vi "Test IV and Ic distribution V3.vi"() -> ()   [LabVIEW 2024]
uses:
  RT fast data.ctl
  <vilib>/LabVIEW Targets/FPGA/cRIO/shared/nicrio_ModuleControls/nicrio_cRIO-9775_RecordDataRates4ChansRing.ctl
  <vilib>/LabVIEW Targets/FPGA/cRIO/shared/nicrio_ModuleControls/nicrio_BasicConversionTime.ctl
  Ramps.ctl
  <resource>/objmgr/ni.dex.rc
  <vilib>/Analysis/NI_AALBase.lvlib
panel:
  in  "Tab Control 2":T1(tab)=enum."Ic distribution"
  out "IV":cluster{"Y":dbl[], "Y":dbl[]}[](graph)
  out "Waveform Graph":dbl[][](graph)
  out "Histogram Graph":T2(graph)={"X Values"=[4.536339111328125, 4.540169677734375, 4.544000244140625, 4.547830810546874, 4.551661376953124, 4.555491943359374, 4.559322509765623, 4.563153076171873, 4.566983642578123, 4.570814208984372, 4.574644775390622, 4.578475341796872, 4.5823059082031214, 4.586136474609371, 4.589967041015621, 4.5937976074218705, 4.59762817382812, 4.60145874023437, 4.6052893066406195, 4.609119873046869, 4.612950439453119, 4.616781005859369, 4.620611572265618, 4.624442138671868, 4.628272705078118, 4.632103271484367, 4.635933837890617, 4.639764404296867, 4.643594970703116, 4.647425537109366, 4.651256103515616, 4.655086669921865, 4.658917236328115, 4.662747802734365, 4.666578369140614, 4.670408935546864, 4.674239501953114, 4.6780700683593635, 4.681900634765613, 4.685731201171863, 4.6895617675781125, 4.693392333984362, 4.697222900390612, 4.7010534667968615, 4.704884033203111, 4.708714599609361, 4.712545166015611, 4.71637573242186, 4.72020629882811, 4.72403686523436, 4.727867431640609, 4.731697998046859, 4.735528564453109, 4.739359130859358, 4.743189697265608, 4.747020263671858, 4.750850830078107, 4.754681396484357, 4.758511962890607, 4.762342529296856, 4.766173095703106, 4.770003662109356, 4.7738342285156055, 4.777664794921855, 4.781495361328105, 4.7853259277343545, 4.789156494140604, 4.792987060546854, 4.7968176269531035, 4.800648193359353, 4.804478759765603, 4.808309326171853, 4.812139892578102, 4.815970458984352, 4.819801025390602, 4.823631591796851, 4.827462158203101, 4.831292724609351, 4.8351232910156, 4.83895385742185, 4.8427844238281, 4.846614990234349, 4.850445556640599, 4.854276123046849, 4.858106689453098, 4.861937255859348, 4.865767822265598, 4.8695983886718475, 4.873428955078097, 4.877259521484347, 4.8810900878905965, 4.884920654296846, 4.888751220703096, 4.8925817871093455, 4.896412353515595, 4.900242919921845, 4.904073486328095, 4.907904052734344, 4.911734619140594, 4.915565185546844], "Histogram: h(x)"=[1, 2, 2, 2, 0, 2, 1, 2, 0, 2, 2, 1, 2, 4, 4, 2, 1, 3, 3, 4, 7, 5, 12, 12, 10, 8, 15, 8, 14, 9, 6, 10, 12, 16, 9, 11, 30, 17, 15, 28, 22, 14, 24, 13, 25, 23, 23, 19, 28, 18, 21, 14, 32, 36, 18, 28, 8, 18, 22, 21, 21, 8, 22, 19, 8, 8, 16, 12, 12, 5, 18, 15, 6, 17, 5, 9, 4, 7, 5, 4, 7, 6, 3, 10, 5, 4, 7, 0, 0, 2, 1, 4, 3, 2, 1, 0, 0, 0, 2, 1]}
  in  "intervals":i32=100
  in  "Tab Control":T3(tab)=enum."Ic"
  in  "cRIO IP":string="//172.22.11.2"
  in  "Data buffer size":i32=1000
  in  "IV parameters":T4={"Records Num"=1, "AI Trigger Configuration"={"Trigger Slope"=enum."Positive", "Trigger Level"=0.89990234375, "Hystesis Value"=0.0, "AI Channel"=0}, "Record PreTrigger Samples"=1, "Record Samples"=2300, "Ic Cut off or curve"=FALSE, "Record Data Rate"=200, "Wait before trigger us"=0, "Cutoff delay usec"=0, "Timing Mode"=enum."High Resolution", "Trigger length ticks"=1, "Timeout"=-1, "Ramps"={"Amp"=8.0, "Delay time 10us"=1000, "Ramp1 time 10us"=1000, "Ramp2 time 10us"=200, "Ramp3 time 10us"=100, "End time 10us"=0}} {"Record Data Rate" items=["20.000 MS/s (NI 9775)"=1, "10.00 MS/s (NI 9775)"=2, "6.667 MS/s (NI 9775)"=3, "5.000 MS/s (NI 9775)"=4, "2.500 MS/s (NI 9775)"=8, "1.667 MS/s (NI 9775)"=12, "1.250 MS/s (NI 9775)"=16, "1.000 MS/s (NI 9775)"=20, "833.333 KS/s (NI 9775)"=24, "714.286 KS/s (NI 9775)"=28, "625.000 KS/s (NI 9775)"=32, "555.556 KS/s (NI 9775)"=36, "500.000 KS/s (NI 9775)"=40, "454.545 KS/s (NI 9775)"=44, "416.667 KS/s (NI 9775)"=48, "384.615 KS/s (NI 9775)"=52, "357.143 KS/s (NI 9775)"=56, "333.333 KS/s (NI 9775)"=60, "312.500 KS/s (NI 9775)"=64, "294.118 KS/s (NI 9775)"=68, "277.778 KS/s (NI 9775)"=72, "263.158 KS/s (NI 9775)"=76, "250.000 KS/s (NI 9775)"=80, "238.095 KS/s (NI 9775)"=84, "227.273 KS/s (NI 9775)"=88, "217.391 KS/s (NI 9775)"=92, "208.333 KS/s (NI 9775)"=96, "200.000 KS/s (NI 9775)"=100, "192.308 KS/s (NI 9775)"=104, "185.185 KS/s (NI 9775)"=108, "178.571 KS/s (NI 9775)"=112, "172.414 KS/s (NI 9775)"=116, "166.667 KS/s (NI 9775)"=120, "161.290 KS/s (NI 9775)"=124, "156.250 KS/s (NI 9775)"=128, "151.515 KS/s (NI 9775)"=132, "147.059 KS/s (NI 9775)"=136, "142.857 KS/s (NI 9775)"=140, "138.889 KS/s (NI 9775)"=144, "135.135 KS/s (NI 9775)"=148, "131.579 KS/s (NI 9775)"=152, "128.205 KS/s (NI 9775)"=156, "125.000 KS/s (NI 9775)"=160, "121.951 KS/s (NI 9775)"=164, "119.048 KS/s (NI 9775)"=168, "116.279 KS/s (NI 9775)"=172, "113.636 KS/s (NI 9775)"=176, "111.111 KS/s (NI 9775)"=180, "108.696 KS/s (NI 9775)"=184, "106.383 KS/s (NI 9775)"=188, "104.167 KS/s (NI 9775)"=192, "102.041 KS/s (NI 9775)"=196, "100.000 KS/s (NI 9775)"=200, "50.000 KS/s (NI 9775)"=400, "33.333 KS/s (NI 9775)"=600, "25.000 KS/s (NI 9775)"=800, "20.000 KS/s (NI 9775)"=1000, "16.667 KS/s (NI 9775)"=1200, "14.286 KS/s (NI 9775)"=1400, "12.500 KS/s (NI 9775)"=1600, "11.111 KS/s (NI 9775)"=1800, "10.000 KS/s (NI 9775)"=2000, "9.091 KS/s (NI 9775)"=2200, "8.333 KS/s (NI 9775)"=2400, "7.692 KS/s (NI 9775)"=2600, "7.143 KS/s (NI 9775)"=2800, "6.667 KS/s (NI 9775)"=3000, "6.250 KS/s (NI 9775)"=3200, "5.882 KS/s (NI 9775)"=3400, "5.556 KS/s (NI 9775)"=3600, "5.000 KS/s (NI 9775)"=4000, "4.762 KS/s (NI 9775)"=4200, "4.545 KS/s (NI 9775)"=4400, "4.348 KS/s (NI 9775)"=4600, "4.167 KS/s (NI 9775)"=4800, "4.000 KS/s (NI 9775)"=5000, "3.846 KS/s (NI 9775)"=5200, "3.571 KS/s (NI 9775)"=5600, "3.333 KS/s (NI 9775)"=6000, "3.125 KS/s (NI 9775)"=6400, "2.941 KS/s (NI 9775)"=6800, "2.778 KS/s (NI 9775)"=7200, "2.632 KS/s (NI 9775)"=7600, "2.500 KS/s (NI 9775)"=8000, "2.381 KS/s (NI 9775)"=8400, "2.273 KS/s (NI 9775)"=8800, "2.174 KS/s (NI 9775)"=9200, "2.083 KS/s (NI 9775)"=9600, "2.000 KS/s (NI 9775)"=10000, "1.923 KS/s (NI 9775)"=10400, "1.852 KS/s (NI 9775)"=10800, "1.786 KS/s (NI 9775)"=11200, "1.724 KS/s (NI 9775)"=11600, "1.667 KS/s (NI 9775)"=12000, "1.613 KS/s (NI 9775)"=12400, "1.563 KS/s (NI 9775)"=12800, "1.515 KS/s (NI 9775)"=13200, "1.471 KS/s (NI 9775)"=13600, "1.429 KS/s (NI 9775)"=14000, "1.389 KS/s (NI 9775)"=14400, "1.351 KS/s (NI 9775)"=14800, "1.316 KS/s (NI 9775)"=15200, "1.282 KS/s (NI 9775)"=15600, "1.250 KS/s (NI 9775)"=16000, "1.220 KS/s (NI 9775)"=16400, "1.190 KS/s (NI 9775)"=16800, "1.163 KS/s (NI 9775)"=17200, "1.136 KS/s (NI 9775)"=17600, "1.111 KS/s (NI 9775)"=18000, "1.087 KS/s (NI 9775)"=18400, "1.064 KS/s (NI 9775)"=18800, "1.042 KS/s (NI 9775)"=19200, "1.020 KS/s (NI 9775)"=19600, "1.000 KS/s (NI 9775)"=20000, "0.980 KS/s (NI 9775)"=20400, "0.962 KS/s (NI 9775)"=20800, "0.943 KS/s (NI 9775)"=21200, "0.926 KS/s (NI 9775)"=21600, "0.909 KS/s (NI 9775)"=22000, "0.893 KS/s (NI 9775)"=22400, "0.877 KS/s (NI 9775)"=22800, "0.862 KS/s (NI 9775)"=23200, "0.847 KS/s (NI 9775)"=23600, "0.833 KS/s (NI 9775)"=24000, "0.820 KS/s (NI 9775)"=24400, "0.806 KS/s (NI 9775)"=24800, "0.794 KS/s (NI 9775)"=25200, "0.781 KS/s (NI 9775)"=25600, "0.694 KS/s (NI 9775)"=28800, "0.625 KS/s (NI 9775)"=32000, "0.568 KS/s (NI 9775)"=35200, "0.521 KS/s (NI 9775)"=38400, "0.446 KS/s (NI 9775)"=44800, "0.391 KS/s (NI 9775)"=51200, "0.347 KS/s (NI 9775)"=57600, "0.313 KS/s (NI 9775)"=64000]}
  in  "Ic parameters":T4={"Records Num"=1000, "AI Trigger Configuration"={"Trigger Slope"=enum."Positive", "Trigger Level"=0.199951171875, "Hystesis Value"=0.0, "AI Channel"=0}, "Record PreTrigger Samples"=1, "Record Samples"=16, "Ic Cut off or curve"=TRUE, "Record Data Rate"=1, "Wait before trigger us"=10000, "Cutoff delay usec"=0, "Timing Mode"=enum."High Resolution", "Trigger length ticks"=1, "Timeout"=-1, "Ramps"={"Amp"=8.0, "Delay time 10us"=1000, "Ramp1 time 10us"=1000, "Ramp2 time 10us"=200, "Ramp3 time 10us"=100, "End time 10us"=0}} {"Record Data Rate" items=["20.000 MS/s (NI 9775)"=1, "10.00 MS/s (NI 9775)"=2, "6.667 MS/s (NI 9775)"=3, "5.000 MS/s (NI 9775)"=4, "2.500 MS/s (NI 9775)"=8, "1.667 MS/s (NI 9775)"=12, "1.250 MS/s (NI 9775)"=16, "1.000 MS/s (NI 9775)"=20, "833.333 KS/s (NI 9775)"=24, "714.286 KS/s (NI 9775)"=28, "625.000 KS/s (NI 9775)"=32, "555.556 KS/s (NI 9775)"=36, "500.000 KS/s (NI 9775)"=40, "454.545 KS/s (NI 9775)"=44, "416.667 KS/s (NI 9775)"=48, "384.615 KS/s (NI 9775)"=52, "357.143 KS/s (NI 9775)"=56, "333.333 KS/s (NI 9775)"=60, "312.500 KS/s (NI 9775)"=64, "294.118 KS/s (NI 9775)"=68, "277.778 KS/s (NI 9775)"=72, "263.158 KS/s (NI 9775)"=76, "250.000 KS/s (NI 9775)"=80, "238.095 KS/s (NI 9775)"=84, "227.273 KS/s (NI 9775)"=88, "217.391 KS/s (NI 9775)"=92, "208.333 KS/s (NI 9775)"=96, "200.000 KS/s (NI 9775)"=100, "192.308 KS/s (NI 9775)"=104, "185.185 KS/s (NI 9775)"=108, "178.571 KS/s (NI 9775)"=112, "172.414 KS/s (NI 9775)"=116, "166.667 KS/s (NI 9775)"=120, "161.290 KS/s (NI 9775)"=124, "156.250 KS/s (NI 9775)"=128, "151.515 KS/s (NI 9775)"=132, "147.059 KS/s (NI 9775)"=136, "142.857 KS/s (NI 9775)"=140, "138.889 KS/s (NI 9775)"=144, "135.135 KS/s (NI 9775)"=148, "131.579 KS/s (NI 9775)"=152, "128.205 KS/s (NI 9775)"=156, "125.000 KS/s (NI 9775)"=160, "121.951 KS/s (NI 9775)"=164, "119.048 KS/s (NI 9775)"=168, "116.279 KS/s (NI 9775)"=172, "113.636 KS/s (NI 9775)"=176, "111.111 KS/s (NI 9775)"=180, "108.696 KS/s (NI 9775)"=184, "106.383 KS/s (NI 9775)"=188, "104.167 KS/s (NI 9775)"=192, "102.041 KS/s (NI 9775)"=196, "100.000 KS/s (NI 9775)"=200, "50.000 KS/s (NI 9775)"=400, "33.333 KS/s (NI 9775)"=600, "25.000 KS/s (NI 9775)"=800, "20.000 KS/s (NI 9775)"=1000, "16.667 KS/s (NI 9775)"=1200, "14.286 KS/s (NI 9775)"=1400, "12.500 KS/s (NI 9775)"=1600, "11.111 KS/s (NI 9775)"=1800, "10.000 KS/s (NI 9775)"=2000, "9.091 KS/s (NI 9775)"=2200, "8.333 KS/s (NI 9775)"=2400, "7.692 KS/s (NI 9775)"=2600, "7.143 KS/s (NI 9775)"=2800, "6.667 KS/s (NI 9775)"=3000, "6.250 KS/s (NI 9775)"=3200, "5.882 KS/s (NI 9775)"=3400, "5.556 KS/s (NI 9775)"=3600, "5.000 KS/s (NI 9775)"=4000, "4.762 KS/s (NI 9775)"=4200, "4.545 KS/s (NI 9775)"=4400, "4.348 KS/s (NI 9775)"=4600, "4.167 KS/s (NI 9775)"=4800, "4.000 KS/s (NI 9775)"=5000, "3.846 KS/s (NI 9775)"=5200, "3.571 KS/s (NI 9775)"=5600, "3.333 KS/s (NI 9775)"=6000, "3.125 KS/s (NI 9775)"=6400, "2.941 KS/s (NI 9775)"=6800, "2.778 KS/s (NI 9775)"=7200, "2.632 KS/s (NI 9775)"=7600, "2.500 KS/s (NI 9775)"=8000, "2.381 KS/s (NI 9775)"=8400, "2.273 KS/s (NI 9775)"=8800, "2.174 KS/s (NI 9775)"=9200, "2.083 KS/s (NI 9775)"=9600, "2.000 KS/s (NI 9775)"=10000, "1.923 KS/s (NI 9775)"=10400, "1.852 KS/s (NI 9775)"=10800, "1.786 KS/s (NI 9775)"=11200, "1.724 KS/s (NI 9775)"=11600, "1.667 KS/s (NI 9775)"=12000, "1.613 KS/s (NI 9775)"=12400, "1.563 KS/s (NI 9775)"=12800, "1.515 KS/s (NI 9775)"=13200, "1.471 KS/s (NI 9775)"=13600, "1.429 KS/s (NI 9775)"=14000, "1.389 KS/s (NI 9775)"=14400, "1.351 KS/s (NI 9775)"=14800, "1.316 KS/s (NI 9775)"=15200, "1.282 KS/s (NI 9775)"=15600, "1.250 KS/s (NI 9775)"=16000, "1.220 KS/s (NI 9775)"=16400, "1.190 KS/s (NI 9775)"=16800, "1.163 KS/s (NI 9775)"=17200, "1.136 KS/s (NI 9775)"=17600, "1.111 KS/s (NI 9775)"=18000, "1.087 KS/s (NI 9775)"=18400, "1.064 KS/s (NI 9775)"=18800, "1.042 KS/s (NI 9775)"=19200, "1.020 KS/s (NI 9775)"=19600, "1.000 KS/s (NI 9775)"=20000, "0.980 KS/s (NI 9775)"=20400, "0.962 KS/s (NI 9775)"=20800, "0.943 KS/s (NI 9775)"=21200, "0.926 KS/s (NI 9775)"=21600, "0.909 KS/s (NI 9775)"=22000, "0.893 KS/s (NI 9775)"=22400, "0.877 KS/s (NI 9775)"=22800, "0.862 KS/s (NI 9775)"=23200, "0.847 KS/s (NI 9775)"=23600, "0.833 KS/s (NI 9775)"=24000, "0.820 KS/s (NI 9775)"=24400, "0.806 KS/s (NI 9775)"=24800, "0.794 KS/s (NI 9775)"=25200, "0.781 KS/s (NI 9775)"=25600, "0.694 KS/s (NI 9775)"=28800, "0.625 KS/s (NI 9775)"=32000, "0.568 KS/s (NI 9775)"=35200, "0.521 KS/s (NI 9775)"=38400, "0.446 KS/s (NI 9775)"=44800, "0.391 KS/s (NI 9775)"=51200, "0.347 KS/s (NI 9775)"=57600, "0.313 KS/s (NI 9775)"=64000]}
  in  "Read point":i32=1
  out "DAQ_CMD_Writer endpoint":refnum<k21>="DAQ_CMD_Writer"
  out "PCreaderI":refnum<k21>="PCreaderI"
  out "PC para writer":refnum<k21>="PCwriter"
  out "DAQ_AI_Reader endpoint":refnum<k21>="DAQ_AI_Reader"
  out "PCreaderV":refnum<k21>="PCreaderV"
  out "error out":errorcluster
  in  "IV length":i32=7500
  in  "IV points start":i32
  out "Time to Init ms":u32=654
  out "Start time ms":u32=3519849804
  in  "Wire resistance":dbl
  out "Done":bool=TRUE
  out "Ic data":dbl[](array[numeric])=[4.69482421875, 4.79443359375, 4.6962890625, 4.82763671875, 4.8427734375, 4.723876953125, 4.7529296875, 4.690673828125, 4.736328125, 4.703125, 4.708740234375, 4.690673828125, 4.791748046875, 4.682373046875, 4.658935546875, 4.798583984375, 4.677001953125, 4.766845703125, 4.741943359375, 4.710205078125, 4.70458984375, 4.718505859375, 4.72802734375, 4.74462890625, 4.757080078125, 4.732177734375, 4.669921875, 4.77783203125, 4.791748046875, 4.740478515625, 4.712890625, 4.802734375, 4.6728515625, 4.710205078125, 4.6962890625, 4.748779296875, 4.7060546875, 4.747314453125, 4.77783203125, 4.6962890625, 4.7294921875, 4.698974609375, 4.7294921875, 4.562255859375, 4.68798828125, 4.610595703125, 4.717041015625, 4.689453125, 4.708740234375, 4.76806640625, 4.67822265625, 4.58154296875, 4.732177734375, 4.7060546875, 4.772216796875, 4.758544921875, 4.772216796875, 4.8525390625, 4.802734375, 4.733642578125, 4.83447265625, 4.8291015625, 4.805419921875, 4.6533203125, 4.69775390625, 4.7626953125, 4.67822265625, 4.72119140625, 4.73486328125, 4.71142578125, 4.75146484375, 4.823486328125, 4.766845703125, 4.755615234375, 4.718505859375, 4.805419921875, 4.773681640625, 4.8330078125, 4.80419921875, 4.72119140625, 4.815185546875, 4.802734375, 4.806884765625, 4.76806640625, 4.91064453125, 4.788818359375, 4.816650390625, 4.806884765625, 4.712890625, 4.758544921875, 4.718505859375, 4.826171875, 4.808349609375, 4.788818359375, 4.732177734375, 4.710205078125, 4.80419921875, 4.763916015625, 4.8095703125, 4.78466796875, 4.780517578125, 4.7294921875, 4.71435546875, 4.736328125, 4.747314453125, 4.779296875, 4.855224609375, 4.78466796875, 4.715576171875, 4.740478515625, 4.7431640625, 4.7763671875, 4.855224609375, 4.741943359375, 4.73486328125, 4.759765625, 4.763916015625, 4.759765625, 4.748779296875, 4.80126953125, 4.77099609375, 4.733642578125, 4.72119140625, 4.73486328125, 4.707275390625, 4.665771484375, 4.69482421875, 4.808349609375, 4.736328125, 4.72802734375, 4.7294921875, 4.765380859375, 4.779296875, 4.750244140625, 4.779296875, 4.65625, 4.668701171875, 4.772216796875, 4.747314453125, 4.723876953125, 4.8857421875, 4.682373046875, 4.71142578125, 4.781982421875, 4.70458984375, 4.77783203125, 4.8291015625, 4.81787109375, 4.7265625, 4.798583984375, 4.8125, 4.8330078125, 4.730712890625, 4.6865234375, 4.808349609375, 4.73779296875, 4.75439453125, 4.78466796875, 4.712890625, 4.790283203125, 4.7294921875, 4.715576171875, 4.736328125, 4.766845703125, 4.723876953125, 4.88427734375, 4.750244140625, 4.715576171875, 4.68115234375, 4.625732421875, 4.69775390625, 4.8193359375, 4.78759765625, 4.740478515625, 4.758544921875, 4.62841796875, 4.632568359375, 4.6796875, 4.7294921875, 4.755615234375, 4.74609375, 4.700439453125, 4.775146484375, 4.725341796875, 4.775146484375, 4.775146484375, 4.669921875, 4.685302734375, 4.70458984375, 4.88427734375, 4.765380859375, 4.717041015625, 4.701904296875, 4.73486328125, 4.75439453125, 4.6533203125, 4.63818359375, 4.6796875, 4.732177734375, 4.675537109375, 4.722412109375, 4.717041015625, 4.733642578125, 4.710205078125, 4.68115234375, 4.72119140625, 4.763916015625, 4.77783203125, 4.68798828125, 4.78466796875, 4.747314453125, 4.73779296875, 4.822021484375, 4.846923828125, 4.859375, 4.733642578125, 4.71435546875, 4.8095703125, 4.855224609375, 4.750244140625, 4.698974609375, 4.739013671875, 4.708740234375, 4.7529296875, 4.718505859375, 4.7431640625, 4.683837890625, 4.685302734375, 4.64501953125, 4.71142578125, 4.81787109375, 4.74609375, 4.730712890625, 4.81103515625, 4.748779296875, 4.682373046875, 4.73779296875, 4.755615234375, 4.66162109375, 4.682373046875, 4.690673828125, 4.77783203125, 4.759765625, 4.76806640625, 4.689453125, 4.8095703125, 4.715576171875, 4.710205078125, 4.6962890625, 4.61474609375, 4.75439453125, 4.617431640625, 4.625732421875, 4.73486328125, 4.62841796875, 4.635498046875, 4.75146484375, 4.74462890625, 4.700439453125, 4.763916015625, 4.66455078125, 4.82080078125, 4.6865234375, 4.765380859375, 4.7431640625, 4.757080078125, 4.7958984375, 4.765380859375, 4.758544921875, 4.690673828125, 4.68798828125, 4.685302734375, 4.74609375, 4.682373046875, 4.70458984375, 4.739013671875, 4.773681640625, 4.674072265625, 4.69482421875, 4.7265625, 4.6728515625, 4.69482421875, 4.76806640625, 4.72802734375, 4.824951171875, 4.7197265625, 4.66162109375, 4.765380859375, 4.71435546875, 4.76123046875, 4.6865234375, 4.750244140625, 4.73779296875, 4.74609375, 4.627197265625, 4.6865234375, 4.736328125, 4.73486328125, 4.723876953125, 4.74462890625, 4.76123046875, 4.587158203125, 4.7060546875, 4.693603515625, 4.73779296875, 4.69775390625, 4.70458984375, 4.72119140625, 4.70458984375, 4.733642578125, 4.6630859375, 4.717041015625, 4.7197265625, 4.864990234375, 4.84130859375, 4.708740234375, 4.701904296875, 4.748779296875, 4.740478515625, 4.775146484375, 4.710205078125, 4.775146484375, 4.750244140625, 4.675537109375, 4.7529296875, 4.74462890625, 4.741943359375, 4.718505859375, 4.6201171875, 4.7197265625, 4.76123046875, 4.755615234375, 4.788818359375, 4.7626953125, 4.816650390625, 4.715576171875, 4.76953125, 4.8525390625, 4.8427734375, 4.80419921875, 4.831787109375, 4.82080078125, 4.8359375, 4.802734375, 4.859375, 4.802734375, 4.773681640625, 4.815185546875, 4.758544921875, 4.89111328125, 4.856689453125, 4.781982421875, 4.848388671875, 4.848388671875, 4.86767578125, 4.91748046875, 4.808349609375, 4.757080078125, 4.798583984375, 4.755615234375, 4.889892578125, 4.765380859375, 4.91064453125, 4.87744140625, 4.781982421875, 4.8525390625, 4.813720703125, 4.889892578125, 4.87744140625, 4.8427734375, 4.849609375, 4.805419921875, 4.88427734375, 4.815185546875, 4.739013671875, 4.838623046875, 4.862060546875, 4.7626953125, 4.79443359375, 4.802734375, 4.747314453125, 4.822021484375, 4.846923828125, 4.733642578125, 4.8525390625, 4.853759765625, 4.797119140625, 4.837158203125, 4.862060546875, 4.816650390625, 4.7197265625, 4.855224609375, 4.732177734375, 4.830322265625, 4.76806640625, 4.759765625, 4.717041015625, 4.730712890625, 4.79296875, 4.790283203125, 4.80126953125, 4.8359375, 4.759765625, 4.7626953125, 4.802734375, 4.722412109375, 4.7763671875, 4.85791015625, 4.76806640625, 4.85791015625, 4.830322265625, 4.797119140625, 4.779296875, 4.78466796875, 4.780517578125, 4.85107421875, 4.8125, 4.800048828125, 4.830322265625, 4.815185546875, 4.815185546875, 4.81103515625, 4.7626953125, 4.788818359375, 4.805419921875, 4.675537109375, 4.89404296875, 4.830322265625, 4.802734375, 4.864990234375, 4.837158203125, 4.740478515625, 4.84130859375, 4.788818359375, 4.864990234375, 4.78759765625, 4.806884765625, 4.765380859375, 4.76806640625, 4.772216796875, 4.67822265625, 4.802734375, 4.798583984375, 4.748779296875, 4.76123046875, 4.73779296875, 4.8095703125, 4.65625, 4.689453125, 4.8095703125, 4.886962890625, 4.79296875, 4.7294921875, 4.76806640625, 4.710205078125, 4.723876953125, 4.747314453125, 4.77099609375, 4.864990234375, 4.600830078125, 4.739013671875, 4.86083984375, 4.748779296875, 4.72119140625, 4.898193359375, 4.701904296875, 4.7431640625, 4.683837890625, 4.783447265625, 4.741943359375, 4.759765625, 4.668701171875, 4.66162109375, 4.6728515625, 4.815185546875, 4.797119140625, 4.692138671875, 4.72119140625, 4.76953125, 4.880126953125, 4.805419921875, 4.8095703125, 4.790283203125, 4.824951171875, 4.71435546875, 4.69775390625, 4.693603515625, 4.77783203125, 4.75439453125, 4.775146484375, 4.7265625, 4.775146484375, 4.739013671875, 4.765380859375, 4.8662109375, 4.775146484375, 4.73779296875, 4.815185546875, 4.7763671875, 4.780517578125, 4.710205078125, 4.747314453125, 4.7529296875, 4.715576171875, 4.798583984375, 4.77783203125, 4.63818359375, 4.63134765625, 4.6865234375, 4.6298828125, 4.690673828125, 4.649169921875, 4.788818359375, 4.72119140625, 4.759765625, 4.6962890625, 4.788818359375, 4.7060546875, 4.732177734375, 4.730712890625, 4.682373046875, 4.693603515625, 4.669921875, 4.642333984375, 4.6796875, 4.64794921875, 4.722412109375, 4.67138671875, 4.669921875, 4.6728515625, 4.68115234375, 4.710205078125, 4.63818359375, 4.723876953125, 4.625732421875, 4.739013671875, 4.6298828125, 4.6796875, 4.667236328125, 4.643798828125, 4.72119140625, 4.683837890625, 4.68115234375, 4.63134765625, 4.739013671875, 4.642333984375, 4.578857421875, 4.712890625, 4.635498046875, 4.6865234375, 4.68798828125, 4.73779296875, 4.650634765625, 4.75439453125, 4.7265625, 4.674072265625, 4.61181640625, 4.60791015625, 4.6298828125, 4.642333984375, 4.61328125, 4.652099609375, 4.736328125, 4.740478515625, 4.6962890625, 4.642333984375, 4.618896484375, 4.700439453125, 4.642333984375, 4.730712890625, 4.6865234375, 4.73486328125, 4.63671875, 4.657470703125, 4.757080078125, 4.660400390625, 4.736328125, 4.723876953125, 4.66455078125, 4.685302734375, 4.692138671875, 4.649169921875, 4.657470703125, 4.610595703125, 4.736328125, 4.710205078125, 4.722412109375, 4.685302734375, 4.71435546875, 4.748779296875, 4.747314453125, 4.823486328125, 4.747314453125, 4.791748046875, 4.76123046875, 4.710205078125, 4.74609375, 4.7958984375, 4.701904296875, 4.6865234375, 4.712890625, 4.740478515625, 4.624267578125, 4.634033203125, 4.67822265625, 4.668701171875, 4.708740234375, 4.6630859375, 4.824951171875, 4.72119140625, 4.6201171875, 4.71435546875, 4.623046875, 4.677001953125, 4.689453125, 4.715576171875, 4.689453125, 4.707275390625, 4.668701171875, 4.732177734375, 4.58984375, 4.718505859375, 4.71435546875, 4.71142578125, 4.67138671875, 4.65478515625, 4.740478515625, 4.73486328125, 4.685302734375, 4.7294921875, 4.7431640625, 4.7197265625, 4.73486328125, 4.84130859375, 4.7265625, 4.635498046875, 4.6865234375, 4.7060546875, 4.722412109375, 4.68798828125, 4.634033203125, 4.674072265625, 4.775146484375, 4.698974609375, 4.74609375, 4.73486328125, 4.67822265625, 4.682373046875, 4.658935546875, 4.730712890625, 4.73486328125, 4.675537109375, 4.7294921875, 4.7431640625, 4.6728515625, 4.69775390625, 4.60498046875, 4.757080078125, 4.674072265625, 4.773681640625, 4.68798828125, 4.740478515625, 4.6796875, 4.780517578125, 4.701904296875, 4.747314453125, 4.779296875, 4.682373046875, 4.712890625, 4.634033203125, 4.747314453125, 4.649169921875, 4.674072265625, 4.674072265625, 4.6796875, 4.66162109375, 4.703125, 4.739013671875, 4.739013671875, 4.73486328125, 4.8193359375, 4.69775390625, 4.64794921875, 4.665771484375, 4.62158203125, 4.625732421875, 4.741943359375, 4.78759765625, 4.73779296875, 4.625732421875, 4.58837890625, 4.68798828125, 4.698974609375, 4.61181640625, 4.6630859375, 4.78759765625, 4.6962890625, 4.772216796875, 4.65478515625, 4.69775390625, 4.718505859375, 4.7265625, 4.73779296875, 4.775146484375, 4.685302734375, 4.700439453125, 4.7060546875, 4.635498046875, 4.717041015625, 4.63671875, 4.739013671875, 4.7060546875, 4.7060546875, 4.700439453125, 4.553955078125, 4.642333984375, 4.634033203125, 4.703125, 4.617431640625, 4.674072265625, 4.6728515625, 4.685302734375, 4.650634765625, 4.715576171875, 4.643798828125, 4.632568359375, 4.63134765625, 4.646484375, 4.80126953125, 4.71435546875, 4.642333984375, 4.7626953125, 4.6865234375, 4.700439453125, 4.682373046875, 4.7197265625, 4.575927734375, 4.701904296875, 4.8095703125, 4.657470703125, 4.674072265625, 4.683837890625, 4.6533203125, 4.692138671875, 4.758544921875, 4.625732421875, 4.7294921875, 4.698974609375, 4.77783203125, 4.72802734375, 4.715576171875, 4.73486328125, 4.733642578125, 4.76123046875, 4.722412109375, 4.68798828125, 4.72119140625, 4.718505859375, 4.7626953125, 4.790283203125, 4.618896484375, 4.69482421875, 4.73779296875, 4.69775390625, 4.710205078125, 4.683837890625, 4.75146484375, 4.798583984375, 4.643798828125, 4.758544921875, 4.657470703125, 4.74462890625, 4.736328125, 4.6728515625, 4.772216796875, 4.617431640625, 4.692138671875, 4.70458984375, 4.63818359375, 4.61474609375, 4.58984375, 4.632568359375, 4.783447265625, 4.692138671875, 4.74462890625, 4.63134765625, 4.69482421875, 4.7197265625, 4.710205078125, 4.730712890625, 4.703125, 4.634033203125, 4.747314453125, 4.667236328125, 4.708740234375, 4.775146484375, 4.59814453125, 4.712890625, 4.683837890625, 4.61181640625, 4.625732421875, 4.592529296875, 4.708740234375, 4.773681640625, 4.57177734375, 4.722412109375, 4.815185546875, 4.63134765625, 4.712890625, 4.76953125, 4.748779296875, 4.62841796875, 4.722412109375, 4.6201171875, 4.652099609375, 4.66455078125, 4.685302734375, 4.677001953125, 4.674072265625, 4.701904296875, 4.677001953125, 4.63818359375, 4.640869140625, 4.73779296875, 4.62841796875, 4.553955078125, 4.617431640625, 4.66455078125, 4.8359375, 4.675537109375, 4.791748046875, 4.717041015625, 4.6728515625, 4.717041015625, 4.63671875, 4.634033203125, 4.657470703125, 4.6630859375, 4.674072265625, 4.66162109375, 4.642333984375, 4.660400390625, 4.5400390625, 4.665771484375, 4.624267578125, 4.62841796875, 4.675537109375, 4.559326171875, 4.650634765625, 4.618896484375, 4.665771484375, 4.603759765625, 4.675537109375, 4.617431640625, 4.63671875, 4.542724609375, 4.599609375, 4.584228515625, 4.5634765625, 4.646484375, 4.546875, 4.587158203125, 4.54833984375, 4.585693359375, 4.642333984375, 4.534423828125, 4.65625, 4.703125, 4.5830078125, 4.646484375, 4.66162109375, 4.6728515625, 4.739013671875, 4.7060546875, 4.7763671875, 4.6533203125, 4.57177734375, 4.6728515625, 4.60498046875, 4.65478515625, 4.57470703125, 4.675537109375, 4.685302734375, 4.682373046875, 4.740478515625, 4.660400390625, 4.669921875, 4.710205078125, 4.61181640625, 4.70458984375, 4.6796875, 4.62158203125, 4.70458984375, 4.624267578125, 4.6201171875, 4.5400390625, 4.63818359375, 4.6962890625, 4.652099609375, 4.665771484375, 4.625732421875, 4.544189453125, 4.68798828125, 4.6865234375, 4.609130859375, 4.66455078125, 4.62158203125, 4.674072265625, 4.593994140625, 4.665771484375, 4.62158203125, 4.618896484375, 4.59130859375, 4.723876953125, 4.7197265625, 4.657470703125, 4.62841796875, 4.68798828125, 4.600830078125, 4.63671875, 4.665771484375, 4.642333984375, 4.741943359375, 4.66455078125, 4.718505859375, 4.658935546875, 4.683837890625, 4.6396484375, 4.68115234375, 4.765380859375, 4.815185546875, 4.674072265625, 4.7529296875, 4.71142578125, 4.646484375, 4.76953125, 4.71142578125, 4.800048828125, 4.733642578125, 4.781982421875, 4.779296875, 4.790283203125, 4.677001953125, 4.79296875, 4.765380859375, 4.69775390625, 4.70458984375, 4.715576171875, 4.7861328125, 4.68798828125, 4.76953125, 4.755615234375, 4.736328125, 4.763916015625, 4.74609375, 4.84130859375, 4.703125, 4.73486328125, 4.71435546875, 4.72802734375, 4.79443359375, 4.690673828125, 4.853759765625, 4.81103515625, 4.698974609375, 4.7626953125, 4.7763671875, 4.715576171875, 4.698974609375, 4.73779296875, 4.725341796875, 4.73779296875, 4.763916015625, 4.802734375, 4.815185546875, 4.822021484375, 4.846923828125, 4.758544921875, 4.757080078125, 4.77099609375, 4.748779296875, 4.76123046875, 4.755615234375, 4.8193359375, 4.85107421875, 4.791748046875, 4.81787109375, 4.86767578125, 4.863525390625, 4.838623046875, 4.8359375, 4.8095703125, 4.822021484375, 4.79443359375, 4.739013671875, 4.816650390625, 4.845458984375, 4.797119140625, 4.75439453125, 4.757080078125]
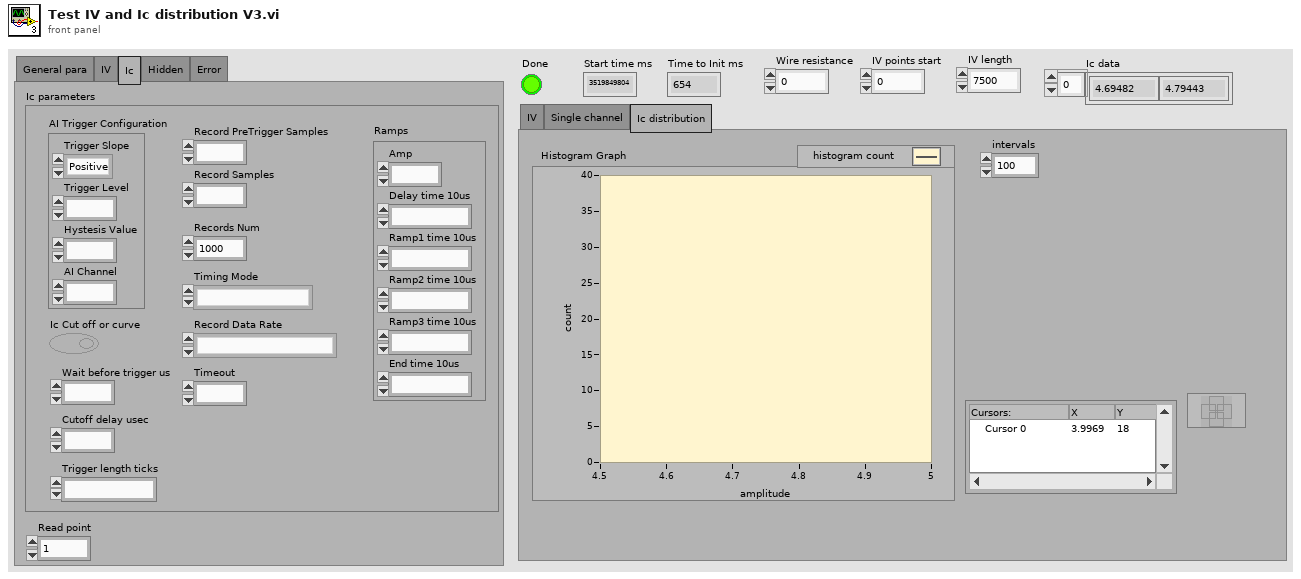
[diagram p1: front panel]
types:
  T1 = enum32{"IV", "Single channel", "Ic distribution"}
  T2 = cluster{"X Values":dbl[], "Histogram: h(x)":i32[]}
  T3 = enum32{"General para", "IV", "Ic", "Hidden", "Error"}
  T4 = typedef "RT fast data.ctl" = cluster{"Records Num":i32, "AI Trigger Configuration":cluster{"Trigger Slope":enum8{"Positive", "Negative"}, "Trigger Level":fxp<+/-,17,5>, "Hystesis Value":fxp<+,16,4>, "AI Channel":u8}, "Record PreTrigger Samples":u32, "Record Samples":u32, "Ic Cut off or curve":bool, "Record Data Rate":T5, "Wait before trigger us":u32, "Cutoff delay usec":u32, "Timing Mode":T6, "Trigger length ticks":u32, "Timeout":i32, "Ramps":T7}
  T5 = typedef "nicrio_cRIO-9775_RecordDataRates4ChansRing.ctl" = u16
  T6 = typedef "nicrio_BasicConversionTime.ctl" = enum8{"High Speed", "High Resolution"}
  T7 = typedef "Ramps.ctl" = cluster{"Amp":fxp<+/-,20,5>, "Delay time 10us":i32, "Ramp1 time 10us":i32, "Ramp2 time 10us":i32, "Ramp3 time 10us":i32, "End time 10us":i32}
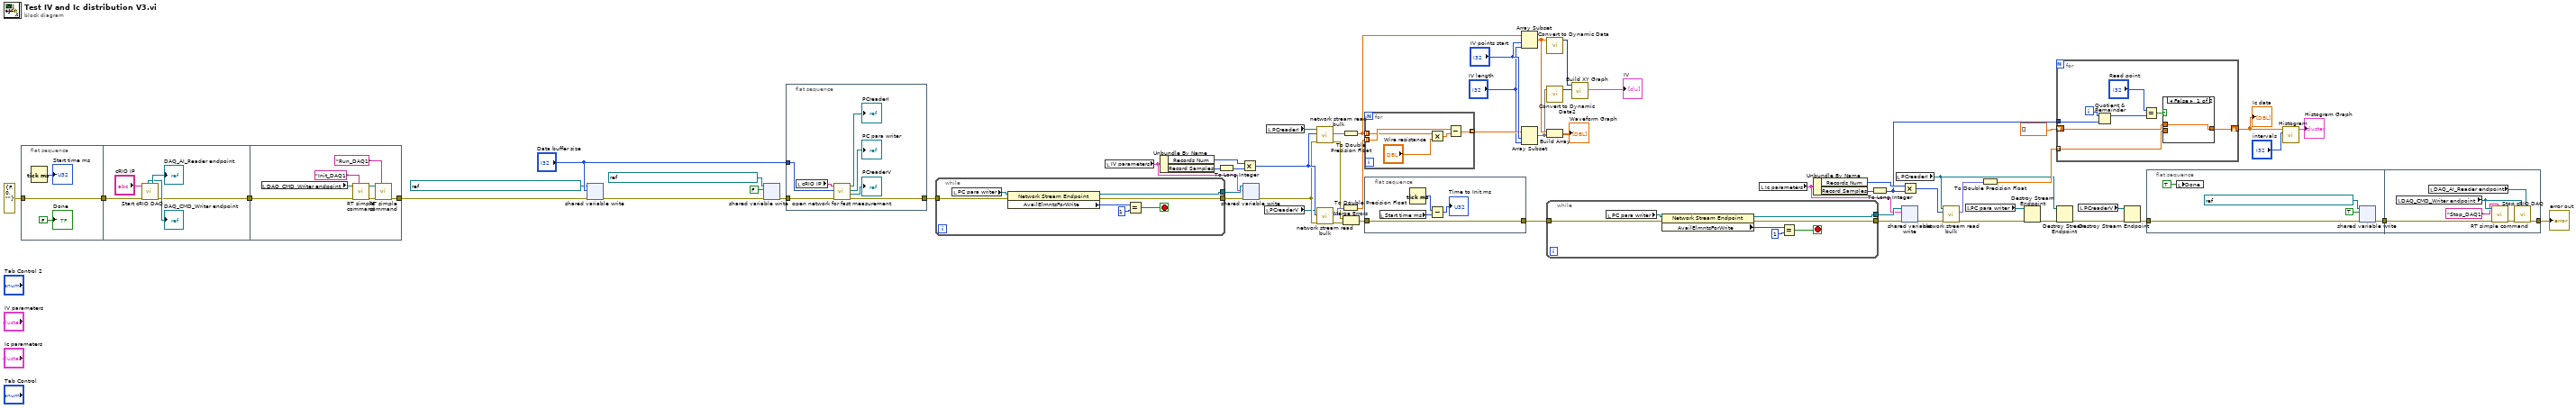
[diagram p0: block diagram]
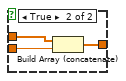
[diagram p2: hidden frame]
diagram:
  n1 = flat-sequence {
    tunnel: errorcluster {"status"=FALSE, "code"=0, "source"=""} ("error in (no error)") -> [w63]
    tunnel: [w63] -> w17
    tunnel: w17 -> [w67]
    tunnel: [w66] -> w7
    tunnel: [w71] -> w16
    tunnel: w7 -> [w76]
    frame #0 {
      n2 = Tick Count (ms)() -> (millisecond timer value=→"Start time ms":u32)
      "Done" <- FALSE ("Done")
    }
    frame #1 {
      n3 = call "Start cRIO DAQ.vi"("error in (no error)"=w67, "cRIO IP"="cRIO IP") -> ("error out"=w66:errorcluster, "DAQ_AI_Reader endpoint"=→"DAQ_AI_Reader endpoint":refnum<k21>, "DAQ_CMD_Writer endpoint"=→"DAQ_CMD_Writer endpoint":refnum<k21>)  [unwired: 7 in]
    }
    frame #2 {
      n4 = local read "DAQ_CMD_Writer endpoint"() -> (w75:refnum<k21>)
      n5 = call "RT simple command.vi"("Command"="Init_DAQ1", "error in (no error)"=w76, "DAQ_CMD_Writer endpoint"=w75) -> ("error out"=w73:errorcluster, "DAQ_CMD_Writer endpoint out"=w72:refnum<k21>)  [unwired: 7 in]
      n6 = call "RT simple command.vi"("Command"="Run_DAQ1", "error in (no error)"=w73, "DAQ_CMD_Writer endpoint"=w72) -> ("error out"=w71:errorcluster)  [unwired: 7 in, 1 out]
    }
  }
  n7 = shared-variable-write(refnum<k21> "ni.var.psp://172.22.11.2/network varibles/Data buffer size" ("shared variable refnum in"), w16, "Data buffer size") -> (w58:errorcluster)  [unwired: 1 out]
  n8 = shared-variable-write(refnum<k21> "ni.var.psp://172.22.11.2/network varibles/RT Stop" ("shared variable refnum in"), w58, FALSE ("RT Stop")) -> (w15:errorcluster)  [unwired: 1 out]
  n9 = flat-sequence {
    tunnel: w15 -> [w83]
    tunnel: "Data buffer size" -> [w82]
    tunnel: [w81] -> w13
    frame #0 {
      n10 = local read "cRIO IP"() -> (w77:string)
      n11 = call "open network for fast measurement.vi"("error in (no error)"=w83, "Data buffer size"=w82, "cRIO IP"=w77) -> ("error out"=w81:errorcluster, "PCreaderV"=→"PCreaderV":refnum<k21>, "PC para writer"=→"PC para writer":refnum<k21>, "PCreaderI"=→"PCreaderI":refnum<k21>)  [unwired: 5 in]
    }
  }
  n12 = while {
    tunnel: w13 -> [w90]
    tunnel: [w86] -> w60
    tunnel: [w85] -> w36
    stop <- w87 stop-if-true
    n13 = local read "PC para writer"() -> (w84:refnum<k21>)
    n14 = property class="Network Stream Endpoint"(reference=w84, error in=w90) -> (reference out=w86:refnum<k21>, error out=w85:errorcluster, "AvailElmntsForWrite"=w89:i32)
    n15 = Equal?(x=w89, y=1) -> (x = y?=w87:bool)
  }
  n16 = local read "IV parameters"() -> (w47:T4)
  n17 = Unbundle By Name(w47) -> ("Records Num"=w46:i32, "Record Samples"=w45:u32)
  n18 = To Long Integer(number=w45) -> (32bit integer=w44:i32)
  n19 = Multiply(x=w46, y=w44) -> (x*y=w31:i32)
  n20 = shared-variable-write(w60, w36, w47) -> (w24:errorcluster)  [unwired: 1 in, 2 out]
  n21 = local read "PCreaderV"() -> (w10:refnum<k21>)
  n22 = local read "PCreaderI"() -> (w11:refnum<k21>)
  n23 = call "network stream read bulk.vi"("endpoint in"=w11, "Data num"=w31, "error in (no error)"=w24) -> ("Data"=w33:fxp<+/-,17,5>[], "error out"=w30:errorcluster)  [unwired: 5 in, 1 out]
  n24 = call "network stream read bulk.vi"("endpoint in"=w10, "Data num"=w31, "error in (no error)"=w24) -> ("Data"=w32:fxp<+/-,17,5>[], "error out"=w29:errorcluster)  [unwired: 5 in, 1 out]
  n25 = To Double Precision Float(number=w32) -> (double precision float=w37:dbl[])
  n26 = Merge Errors(w30, w29) -> (w35:errorcluster)
  n27 = To Double Precision Float(number=w33) -> (double precision float=w22:dbl[])
  n28 = for {
    tunnel: w37 -> [w95] mode=indexing
    tunnel: w22 -> [w93] mode=indexing
    tunnel: [w91] -> w21 mode=indexing
    n29 = Multiply(x=w93, y="Wire resistance") -> (x*y=w92:dbl)
    n30 = Subtract(x=w95, y=w92) -> (x-y=w91:dbl)
  }
  n31 = flat-sequence {
    tunnel: w35 -> [w96]
    tunnel: [w96] -> w34
    frame #0 {
      n32 = local read "Start time ms"() -> (w98:u32)
      n33 = Tick Count (ms)() -> (millisecond timer value=w99:u32)
      n34 = Subtract(x=w99, y=w98) -> (x-y=→"Time to Init ms":u32)
    }
  }
  n35 = Array Subset(array=w22, index="IV points start", length="IV length") -> (w6:dbl[])
  n36 = Array Subset(array=w21, index="IV points start", length="IV length") -> (w5:dbl[])
  n37 = call "Convert to Dynamic Data"("Array"=w6) -> ("Dynamic Data Type"=w52:dynamicdata)  [unwired: 3 in]
  n38 = call "Convert to Dynamic Data2"("Array"=w5) -> ("Dynamic Data Type"=w51:dynamicdata)  [unwired: 3 in]
  n39 = Build Array(w6, w5) -> (→"Waveform Graph":dbl[][])
  n40 = while {
    tunnel: w34 -> [w104]
    tunnel: [w102] -> w55
    tunnel: [w101] -> w54
    stop <- w103 stop-if-true
    n41 = local read "PC para writer"() -> (w100:refnum<k21>)
    n42 = property class="Network Stream Endpoint"(reference=w100, error in=w104) -> (reference out=w102:refnum<k21>, error out=w101:errorcluster, "AvailElmntsForWrite"=w106:i32)
    n43 = Equal?(x=w106, y=1) -> (x = y?=w103:bool)
  }
  n44 = call "Build XY Graph"("Y Input"=w51, "X Input"=w52) -> ("XY Graph"=→"IV":cluster{"X":dbl[], "Y":dbl[]}[])  [unwired: 8 in, 1 out]
  n45 = local read "Ic parameters"() -> (w50:T4)
  n46 = Unbundle By Name(w50) -> ("Records Num"=w49:i32, "Record Samples"=w48:u32)
  n47 = To Long Integer(number=w48) -> (32bit integer=w41:i32)
  n48 = local read "PCreaderI"() -> (w9:refnum<k21>)
  n49 = shared-variable-write(w55, w54, w50) -> (w27:errorcluster)  [unwired: 1 in, 2 out]
  n50 = Multiply(x=w49, y=w41) -> (x*y=w25:i32)
  n51 = call "network stream read bulk.vi"("endpoint in"=w9, "Data num"=w25, "error in (no error)"=w27) -> ("Data"=w28:fxp<+/-,17,5>[], "error out"=w26:errorcluster)  [unwired: 5 in, 1 out]
  n52 = local read "PC para writer"() -> (w12:refnum<k21>)
  n53 = To Double Precision Float(number=w28) -> (double precision float=w42:dbl[])
  n54 = Destroy Stream Endpoint(8:w26, 11:w12) -> (0:w59:errorcluster)
  n55 = for {
    tunnel: w42 -> [w108] mode=indexing
    tunnel: w41 -> [w114]
    shift-right: [w110] -> w39
    shift-left: dbl[] [] -> [w109]
    i -> [w113]
    n56 = Quotient & Remainder(x=w113, y=w114) -> (x-y*floor(x/y)=w112:i32)  [unwired: 1 out]
    n57 = Equal?(x="Read point", y=w112) -> (x = y?=w107:bool)
    n58 = case shown="False" w107 {
      tunnel: [w115 w118] -> w110
      tunnel: w109 -> [w115 w117]
      tunnel: w108 -> [_ w116]
      frame False {
      }
      frame True {
        n59 = Build Array (concatenate)(w117, w116) -> (w118:dbl[])
      }
    }
  }
  "Ic data" <- w39
  n60 = Destroy Stream Endpoint(8:w59, 11:w9) -> (0:w57:errorcluster)
  n61 = local read "PCreaderV"() -> (w8:refnum<k21>)
  n62 = Destroy Stream Endpoint(8:w57, 11:w8) -> (0:w56:errorcluster)
  n63 = flat-sequence {
    tunnel: w56 -> [w122]
    tunnel: [w123] -> w19
    tunnel: w19 -> [w127]
    tunnel: [w128] -> w18
    frame #0 {
      n64 = local write "Done"(TRUE ("Done")) -> ()
      n65 = shared-variable-write(refnum<k21> "ni.var.psp://172.22.11.2/network varibles/RT Stop" ("shared variable refnum in"), w122, TRUE ("RT Stop")) -> (w123:errorcluster)  [unwired: 1 out]
    }
    frame #1 {
      n66 = local read "DAQ_CMD_Writer endpoint"() -> (w125:refnum<k21>)
      n67 = local read "DAQ_AI_Reader endpoint"() -> (w129:refnum<k21>)
      n68 = call "RT simple command.vi"("Command"="Stop_DAQ1", "error in (no error)"=w127, "DAQ_CMD_Writer endpoint"=w125) -> ("error out"=w126:errorcluster)  [unwired: 7 in, 1 out]
      n69 = call "Stop cRIO DAQ.vi"("DAQ_AI_Reader endpoint"=w129, "DAQ_CMD_Writer endpoint"=w125, "error in (no error)"=w126) -> ("error out"=w128:errorcluster)  [unwired: 8 in]
    }
  }
  n70 = call <vilib>:"Histogram.vi"("intervals"="intervals", "X"=w39) -> ("Histogram Graph"=→"Histogram Graph":T2)  [unwired: 6 in, 3 out]
  "error out" <- w18
